vi "evo irimager set temperature range.vi"(10 "t_max":i32, 11 "t_min":i32) -> (3 "function return":i32)   [LabVIEW 2017, in "libirimager_direct_binding.lvlib"]
doc: "DIRECT_API int evo_irimager_set_temperature_range(int t_min, int t_max);"
uses:
  libirimager_direct_binding.lvlib
  labview/libirimager.dll
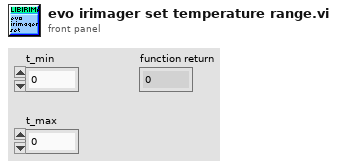
[diagram p1: front panel]
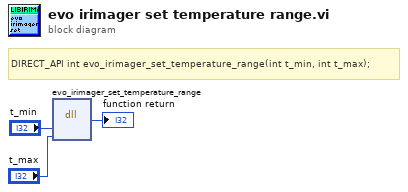
[diagram p0: block diagram]
diagram:
  # "DIRECT_API int evo_irimager_set_temperature_range(int t_min, int t_max);"
  n1 = dll-call lib="C:/Users/HelmutEngelhardt/Documents/labview/libirimager.dll" fn="evo_irimager_set_temperature_range"("t_min"="t_min", "t_max"="t_max") -> ("Rückgabetyp"=→"function return":i32)  [unwired: 5 in, 2 out]
